vi "Final.vi"() -> ()   [LabVIEW 2022 SP3]
uses:
  <vilib>/DAQmx/read.llb/DAQmx Read (Analog 1D DBL NChan 1Samp).vi
  <vilib>/DAQmx/write.llb/DAQmx Write (Digital Bool 1Line 1Point).vi
  <vilib>/DAQmx/create/channels.llb/DAQmx Create Channel (DO-Digital Output).vi
  <vilib>/DAQmx/create/channels.llb/DAQmx Create Channel (AI-Voltage-Basic).vi
  <vilib>/DAQmx/miscellaneous.llb/DAQmx Fill In Error Info.vi
panel:
  out "Thermometer":dbl(slide) scale=0.0..60.0
  in  "VISA resource name":refnum<visa-resource-name>
  out "Iteration CH2":dbl
  in  "LDR Bridge Voltage (Auto)":dbl
  out "Detection State":dbl
  out "People Count":dbl
  out "AI 3":dbl
  out "AI 2":dbl
  out "AI 1":dbl
  in  "Analog Inputs":tag
  in  "Fan Output":tag
  out "Fan Speed Level":dbl
  out "Fan State":bool
  out "Temp Sensor Input Value":dbl
  out "Temperature in *C":ext format="%0.5f"
  in  "LED Output":tag
  out "Light Intensity Level":dbl
  in  "Existance":bool
  in  "Loop Breaker 1":bool
  out "Leaving Trigger":bool
  out "EnteringTrigger":bool
  in  "Loop Breaker 2":bool
  out "LDR Input Value":dbl
  # "Input & Output Channels"
  # "Sensor Readings"
  # "Lighting System"
  # "Temperature Sensor \nReading"
  # "LDR Bridge Voltage"
  # "LDR Input Value"
  # "People Counter"
  # "Cooling System"
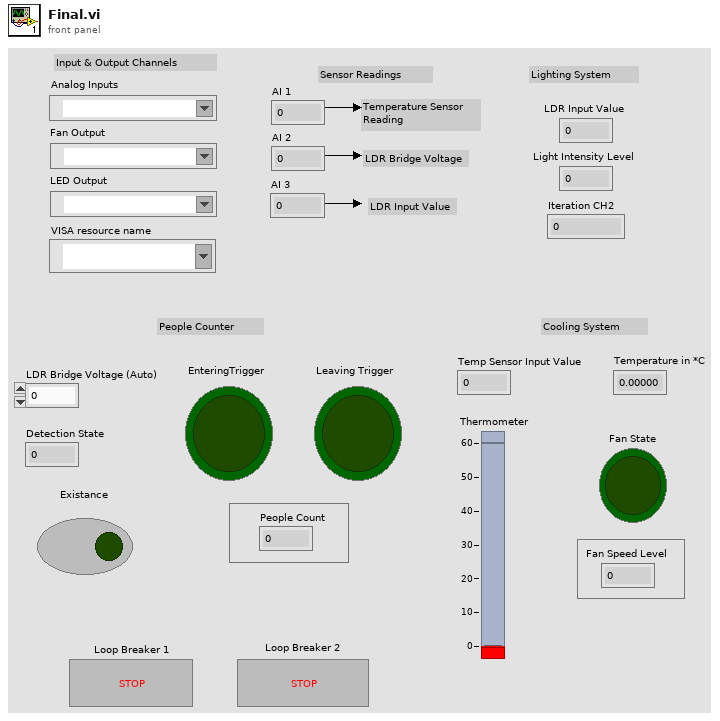
[diagram p1: front panel]
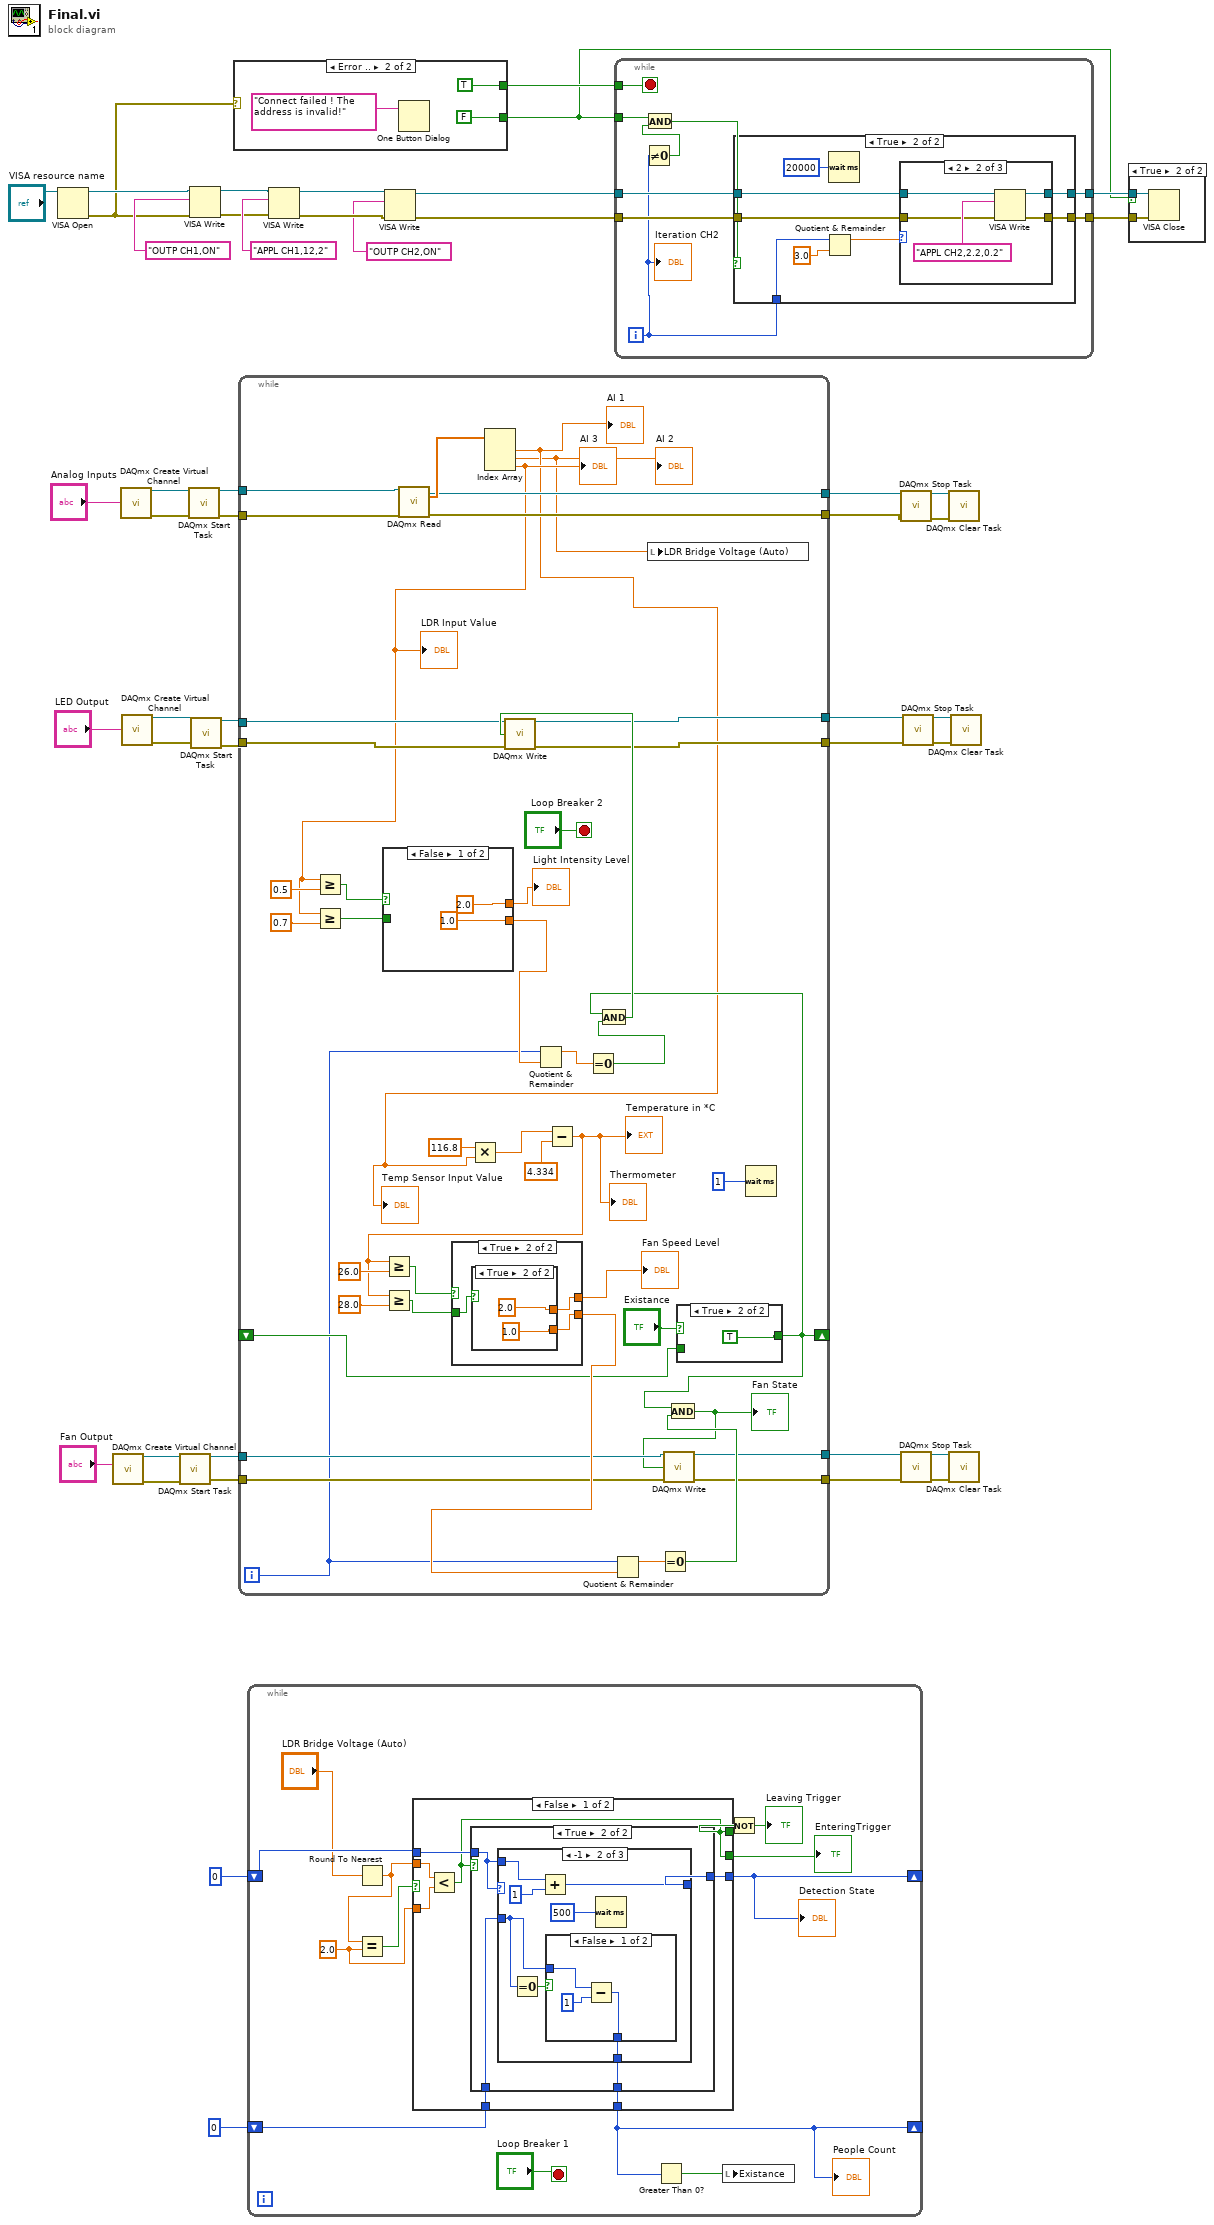
[diagram p0: block diagram]
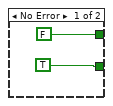
[diagram p3: hidden frame]
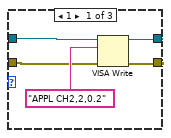
[diagram p5: hidden frame]
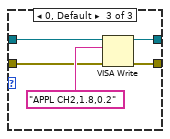
[diagram p6: hidden frame]
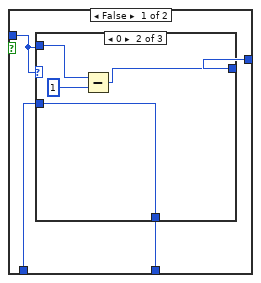
[diagram p7: hidden frame]
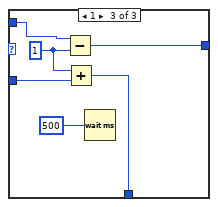
[diagram p9: hidden frame]
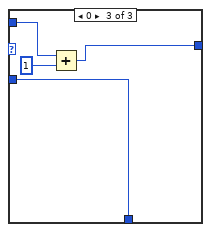
[diagram p12: hidden frame]
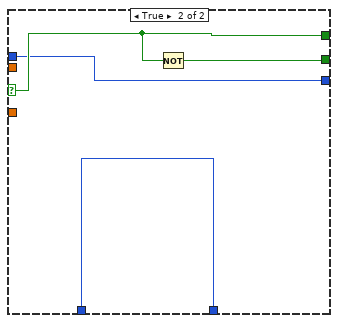
[diagram p13: hidden frame]
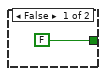
[diagram p14: hidden frame]
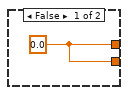
[diagram p15: hidden frame]
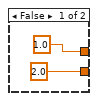
[diagram p16: hidden frame]
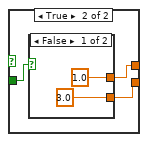
[diagram p17: hidden frame]
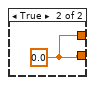
[diagram p18: hidden frame]
diagram:
  n1 = VISA Open(VISA resource name="VISA resource name") -> (VISA resource name=w12:refnum<visa-resource-name>, error out=w11:errorcluster)  [unwired: 4 in]
  n2 = call-poly <vilib>:"DAQmx Create Virtual Channel.vi"("lines"="Fan Output") -> ("task out"=w34:refnum<k21>, "error out"=w33:errorcluster)  [unwired: 13 in]
  n3 = call-poly <vilib>:"DAQmx Create Virtual Channel.vi"("physical channels"="Analog Inputs") -> ("task out"=w26:refnum<k21>, "error out"=w25:errorcluster)  [unwired: 13 in]
  n4 = call-poly <vilib>:"DAQmx Create Virtual Channel.vi"("lines"="LED Output") -> ("task out"=w45:refnum<k21>, "error out"=w44:errorcluster)  [unwired: 13 in]
  n5 = call <vilib>:"DAQmx Start Task.vi"("task/channels in"=w34, "error in"=w33) -> ("task out"=w31:refnum<k21>, "error out"=w30:errorcluster)  [unwired: 12 in]
  n6 = call <vilib>:"DAQmx Start Task.vi"("task/channels in"=w26, "error in"=w25) -> ("task out"=w24:refnum<k21>, "error out"=w23:errorcluster)  [unwired: 12 in]
  n7 = VISA Write(VISA resource name=w12, write buffer="OUTP CH1,ON", error in (no error)=w11) -> (VISA resource name out=w15:refnum<visa-resource-name>, error out=w10:errorcluster)  [unwired: 1 out]
  n8 = call <vilib>:"DAQmx Start Task.vi"("task/channels in"=w45, "error in"=w44) -> ("task out"=w43:refnum<k21>, "error out"=w42:errorcluster)  [unwired: 12 in]
  n9 = case shown="Error .." w11 {
    tunnel: [FALSE TRUE] -> w2
    tunnel: [TRUE FALSE] -> w1
    frame No Error {
    }
    frame Error {
      n10 = One Button Dialog(message="Connect failed ! The address is invalid!") -> ()  [unwired: 1 in, 1 out]
    }
  }
  n11 = while {
    tunnel: w43 -> [w83]
    tunnel: w42 -> [w82]
    tunnel: [w61] -> w39
    tunnel: [w84] -> w38
    tunnel: w31 -> [w70]
    tunnel: w30 -> [w69]
    tunnel: [w68] -> w29
    tunnel: [w67] -> w28
    tunnel: w24 -> [w66]
    tunnel: w23 -> [w65]
    tunnel: [w63] -> w20
    tunnel: [w62] -> w18
    shift-right: [w57] -> _
    shift-left: _ -> [w58]
    i -> [w54]
    stop <- "Loop Breaker 2" stop-if-true
    n12 = call-poly <vilib>:"DAQmx Read.vi"("task/channels in"=w66, "error in"=w65) -> ("task out"=w63:refnum<k21>, "data"=w64:dbl[], "error out"=w62:errorcluster)  [unwired: 11 in]
    n13 = Index Array(array=w64) -> (element #1=w56:dbl, element #2=w55:dbl, element #3=w60:dbl)  [unwired: 3 in]
    "LDR Input Value" <- w60
    "Temp Sensor Input Value" <- w56
    "AI 1" <- w56
    "AI 2" <- w55
    "AI 3" <- w60
    n14 = Greater Or Equal?(x=w60, y=0.5) -> (x >= y?=w88:bool)
    n15 = Greater Or Equal?(x=w60, y=0.7) -> (x >= y?=w87:bool)
    n16 = case shown="False" w88 {
      tunnel: [2.0 ("y") w107] -> w86
      tunnel: w87 -> [_ w109]
      tunnel: [1.0 ("y") w108] -> w85
      frame False {
      }
      frame True {
        n17 = case shown="False" w109 {
          tunnel: [1.0 ("y") w112] -> w107
          tunnel: [3.0 ("y") w112] -> w108
          frame False {
          }
          frame True {
            w112 = 0.0 ("y")
          }
        }
      }
    }
    "Light Intensity Level" <- w86
    n18 = Multiply(x=116.8 ("y"), y=w56) -> (x*y=w80:dbl)
    n19 = Quotient & Remainder(x=w54, y=w85) -> (x-y*floor(x/y)=w93:dbl)  [unwired: 1 out]
    n20 = Subtract(x=w80, y=4.334) -> (x-y=w52:dbl)
    "Temperature in *C" <- w52
    "Thermometer" <- w52
    n21 = Greater Or Equal?(x=w52, y=26.0) -> (x >= y?=w74:bool)
    n22 = Greater Or Equal?(x=w52, y=28.0) -> (x >= y?=w73:bool)
    n23 = case shown="True" w74 {
      tunnel: [w97 w98] -> w72
      tunnel: w73 -> [_ w100]
      tunnel: [w97 w99] -> w71
      frame False {
        w97 = 0.0 ("y")
      }
      frame True {
        n24 = case shown="True" w100 {
          tunnel: [1.0 ("y") 2.0 ("y")] -> w98
          tunnel: [2.0 ("y") 1.0 ("y")] -> w99
          frame False {
          }
          frame True {
          }
        }
      }
    }
    "Fan Speed Level" <- w72
    n25 = Equal To 0?(x=w93) -> (x = 0?=w92:bool)
    n26 = Quotient & Remainder(x=w54, y=w71) -> (x-y*floor(x/y)=w78:dbl)  [unwired: 1 out]
    n27 = local write "LDR Bridge Voltage (Auto)"(w55) -> ()
    n28 = Equal To 0?(x=w78) -> (x = 0?=w77:bool)
    n29 = case shown="True" "Existance" {
      tunnel: [FALSE TRUE] -> w57
      tunnel: w58 -> [_ _]
      frame False {
      }
      frame True {
      }
    }
    n30 = And(x=w57, y=w92) -> (x .and. y?=w91:bool)
    n31 = call-poly <vilib>:"DAQmx Write.vi"("task/channels in"=w83, "data"=w91, "error in"=w82) -> ("task out"=w61:refnum<k21>, "error out"=w84:errorcluster)  [unwired: 10 in, 1 out]
    n32 = And(x=w57, y=w77) -> (x .and. y?=w53:bool)
    "Fan State" <- w53
    n33 = call-poly <vilib>:"DAQmx Write.vi"("task/channels in"=w70, "data"=w53, "error in"=w69) -> ("task out"=w68:refnum<k21>, "error out"=w67:errorcluster)  [unwired: 10 in, 1 out]
    n34 = Wait (ms)(milliseconds to wait=u32 1) -> ()  [unwired: 1 out]
  }
  n35 = while {
    shift-right: [w117] -> _
    shift-left: i16 0 ("y") -> [w124]
    shift-right: [w114] -> _
    shift-left: i16 0 ("y") -> [w115]
    stop <- "Loop Breaker 1" stop-if-true
    w121 = 2.0 ("x")
    n36 = Round To Nearest(number="LDR Bridge Voltage (Auto)") -> (nearest integer value=w120:dbl)
    n37 = Equal?(x=w120, y=w121) -> (x = y?=w123:bool)
    n38 = case shown="False" w123 {
      selector: w123 -> [_ w173]
      tunnel: w124 -> [w130 w172]
      tunnel: w120 -> [w132 _]
      tunnel: w121 -> [w131 _]
      tunnel: [w128 w172] -> w117
      tunnel: [w129 w173] -> w118
      tunnel: [w129 w170] -> w119
      tunnel: w115 -> [w126 w171]
      tunnel: [w127 w171] -> w114
      frame False {
        n39 = Less?(x=w132, y=w131) -> (x < y?=w129:bool)
        n40 = case shown="True" w129 {
          tunnel: w130 -> [w135 w152]
          tunnel: [w136 w150] -> w128
          tunnel: [w134 w151] -> w127
          tunnel: w126 -> [w133 w149]
          frame False {
            n41 = case shown="0" w135 {
              tunnel: w135 -> [w138 w140 w147]
              tunnel: [w138 w142 w148] -> w136
              tunnel: w133 -> [w137 w139 w146]
              tunnel: [w137 w139 w144] -> w134
              frame -1, Default {
              }
              frame 0 {
                n42 = Subtract(x=w140, y=i16 1) -> (x-y=w142:i16)
              }
              frame 1 {
                w145 = i16 1 ("y")
                n43 = Subtract(x=w147, y=w145) -> (x-y=w148:i16)
                n44 = Add(x=w145, y=w146) -> (x+y=w144:i16)
                n45 = Wait (ms)(milliseconds to wait=u32 500) -> ()  [unwired: 1 out]
              }
            }
          }
          frame True {
            n46 = case shown="-1" w152 {
              tunnel: w152 -> [w154 w160 w167]
              tunnel: [w154 w161 w168] -> w150
              tunnel: w149 -> [w153 w156 w166]
              tunnel: [w153 w157 w166] -> w151
              frame 1, Default {
              }
              frame -1 {
                n47 = Equal To 0?(x=w156) -> (x = 0?=w158:bool)
                n48 = Add(x=w160, y=i16 1) -> (x+y=w161:i16)
                n49 = case shown="False" w158 {
                  tunnel: [w162 w165] -> w157
                  tunnel: w156 -> [w164 w165]
                  frame False {
                    n50 = Subtract(x=w164, y=i16 1) -> (x-y=w162:i16)
                  }
                  frame True {
                  }
                }
                n51 = Wait (ms)(milliseconds to wait=u32 500) -> ()  [unwired: 1 out]
              }
              frame 0 {
                n52 = Add(x=w167, y=i16 1) -> (x+y=w168:i16)
              }
            }
          }
        }
      }
      frame True {
        n53 = Not(x=w173) -> (.not. x?=w170:bool)
      }
    }
    "EnteringTrigger" <- w119
    "People Count" <- w114
    "Detection State" <- w117
    n54 = Greater Than 0?(x=w114) -> (x > 0?=w116:bool)
    n55 = local write "Existance"(w116) -> ()
    n56 = Not(x=w118) -> (.not. x?=→"Leaving Trigger":bool)
  }
  n57 = VISA Write(VISA resource name=w15, write buffer="APPL CH1,12,2", error in (no error)=w10) -> (VISA resource name out=w5:refnum<visa-resource-name>, error out=w4:errorcluster)  [unwired: 1 out]
  n58 = VISA Write(VISA resource name=w5, write buffer="OUTP CH2,ON", error in (no error)=w4) -> (VISA resource name out=w7:refnum<visa-resource-name>, error out=w6:errorcluster)  [unwired: 1 out]
  n59 = while {
    tunnel: w7 -> [w182]
    tunnel: [w179] -> w8
    tunnel: [w178] -> w9
    tunnel: w6 -> [w177]
    tunnel: w1 -> [w176]
    tunnel: w2 -> [w175]
    i -> [w174]
    stop <- w175 stop-if-true
    n60 = Not Equal To 0?(x=w174) -> (x != 0?=w180:bool)
    n61 = And(x=w176, y=w180) -> (x .and. y?=w181:bool)
    n62 = case shown="True" w181 {
      tunnel: w182 -> [w184 w186]
      tunnel: w174 -> [_ w191]
      tunnel: [w184 w189] -> w179
      tunnel: w177 -> [w183 w185]
      tunnel: [w183 w188] -> w178
      frame False {
      }
      frame True {
        n63 = Quotient & Remainder(x=w191, y=3.0) -> (x-y*floor(x/y)=w187:dbl)  [unwired: 1 out]
        n64 = Wait (ms)(milliseconds to wait=u32 20000) -> ()  [unwired: 1 out]
        n65 = case shown="2" w187 {
          tunnel: [w196 w201 w206] -> w189
          tunnel: [w195 w200 w205] -> w188
          tunnel: w185 -> [w194 w199 w204]
          tunnel: w186 -> [w193 w198 w203]
          frame 1 {
            n66 = VISA Write(VISA resource name=w193, write buffer="APPL CH2,2,0.2", error in (no error)=w194) -> (VISA resource name out=w196:refnum<visa-resource-name>, error out=w195:errorcluster)  [unwired: 1 out]
          }
          frame 2 {
            n67 = VISA Write(VISA resource name=w198, write buffer="APPL CH2,2.2,0.2", error in (no error)=w199) -> (VISA resource name out=w201:refnum<visa-resource-name>, error out=w200:errorcluster)  [unwired: 1 out]
          }
          frame 0, Default {
            n68 = VISA Write(VISA resource name=w203, write buffer="APPL CH2,1.8,0.2", error in (no error)=w204) -> (VISA resource name out=w206:refnum<visa-resource-name>, error out=w205:errorcluster)  [unwired: 1 out]
          }
        }
      }
    }
    "Iteration CH2" <- w174
  }
  n69 = call <vilib>:"DAQmx Stop Task.vi"("task/channels in"=w20, "error in"=w18) -> ("task out"=w22:refnum<k21>, "error out"=w21:errorcluster)  [unwired: 12 in]
  n70 = call <vilib>:"DAQmx Stop Task.vi"("task/channels in"=w29, "error in"=w28) -> ("task out"=w36:refnum<k21>, "error out"=w35:errorcluster)  [unwired: 12 in]
  n71 = call <vilib>:"DAQmx Stop Task.vi"("task/channels in"=w39, "error in"=w38) -> ("task out"=w41:refnum<k21>, "error out"=w40:errorcluster)  [unwired: 12 in]
  n72 = call <vilib>:"DAQmx Clear Task.vi"("task in"=w22, "error in"=w21) -> ()  [unwired: 13 in, 1 out]
  n73 = call <vilib>:"DAQmx Clear Task.vi"("task in"=w36, "error in"=w35) -> ()  [unwired: 13 in, 1 out]
  n74 = call <vilib>:"DAQmx Clear Task.vi"("task in"=w41, "error in"=w40) -> ()  [unwired: 13 in, 1 out]
  n75 = case shown="True" w1 {
    tunnel: w9 -> [_ w209]
    tunnel: w8 -> [_ w208]
    frame False {
    }
    frame True {
      n76 = VISA Close(VISA resource name=w208, error in (no error)=w209) -> ()  [unwired: 1 out]
    }
  }
